vi "binary to gray.vi"() -> ()   [LabVIEW 2020]
panel:
  out "G4":bool
  out "G3":bool
  out "G2":bool
  out "G1":bool
  in  "B4":bool
  in  "B3":bool
  in  "B2":bool
  in  "B1":bool
  # "4 Bit Binary input to Gray Output"
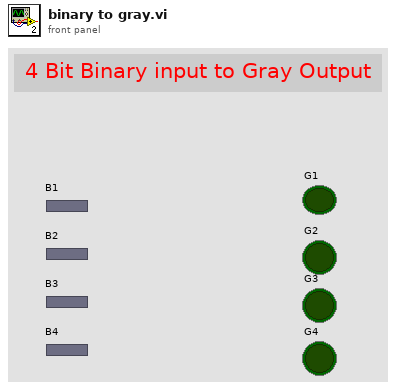
[diagram p1: front panel]
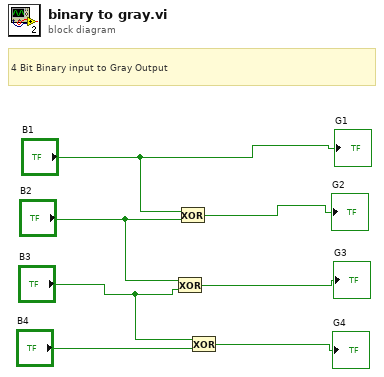
[diagram p0: block diagram]
diagram:
  # "4 Bit Binary input to Gray Output"
  n1 = Exclusive Or(1:"B3", 2:"B2") -> (0:→"G3":bool)
  n2 = Exclusive Or(1:"B2", 2:"B1") -> (0:→"G2":bool)
  n3 = Exclusive Or(1:"B4", 2:"B3") -> (0:→"G4":bool)
  "G1" <- "B1"
